vi "AlGaAs_SL_v09.vi"(2 "Debug Mode":bool, 3 "Elapsed Time(s)":dbl, 4 "State":enum16{"Edit", "Start", "Run", "End", "Idle"}(ring), 5 "Argument List In":string[](array[string])) -> (0 "Status Out":string, 1 "Argument List Out":string[](array[string]))   [LabVIEW 2011]
panel:
  out "tPeriod(s)":dbl
  in  "nPeriods":dbl
  out "time array":dbl[](array[numeric])
  out "nPeriod":dbl
  out "tTotal(s) 2":dbl
  out "is_OK":bool
  out "tTotal(s)":dbl
  in  "Tab Control":enum32{"Step 1", "Step 2", "Step 3", "Step 4"}(tab)
  in  "run Ga 1":bool caption="run Ga"
  in  "run Al 1":bool caption="run Al"
  in  "Al flow 1":dbl caption="Al flow(0-100sccm)" format="%.1f"
  in  "time 1":dbl caption="time(s)"
  in  "Ga flow 1":dbl caption="Ga flow(0-10sccm)" format="%.3f"
  in  "run Ga 2":bool caption="run Ga"
  in  "run Al 2":bool caption="run Al"
  in  "Al flow 2":dbl caption="Al flow (0-100sccm)" format="%.1f"
  in  "Ga flow 2":dbl caption="Ga flow (0-10sccm)" format="%.3f"
  in  "time 2":dbl caption="time(s)"
  in  "time 3":dbl caption="time(s)"
  in  "Al flow 3":dbl caption="Al flow (0-100sccm)" format="%.1f"
  in  "run Al 3":bool caption="run Al"
  in  "Ga flow 3":dbl caption="Ga flow (0-10sccm)" format="%.3f"
  in  "run Ga 3":bool caption="run Ga"
  in  "time 4":dbl caption="time(s)"
  in  "Al flow 4":dbl caption="Al flow (0-100sccm)" format="%.1f"
  in  "run Al 4":bool caption="run Al"
  in  "Ga flow 4":dbl caption="Ga flow (0-10sccm)" format="%.3f"
  in  "run Ga 4":bool caption="run Ga"
  out "tphase(s)":dbl[](array[numeric])
  out "phase":i32
  in  "Cancel":bool
  in  "OK":bool
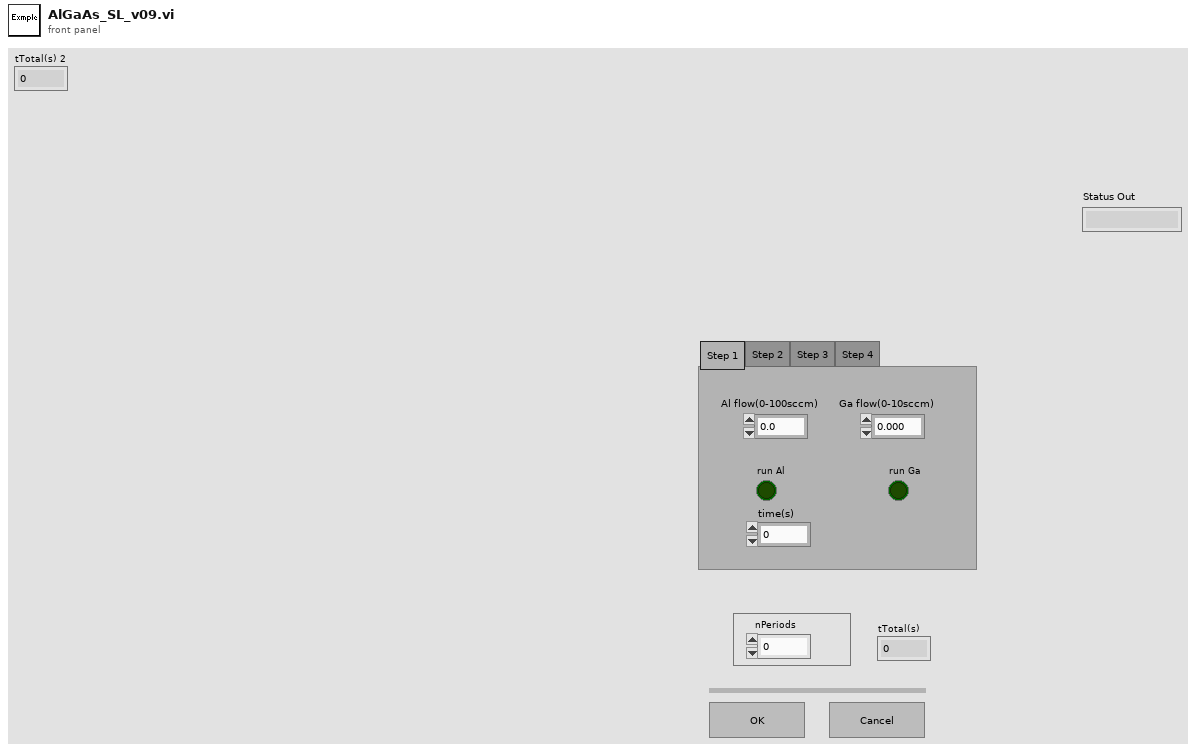
[diagram p1: front panel]
types:
  T1 = enum16{"Discrete", "Continuous", "Instantaneous"}
  T2 = enum32{"Invalid", "Default", "Floating", "Floating/Auto-Hide", "Modal"}
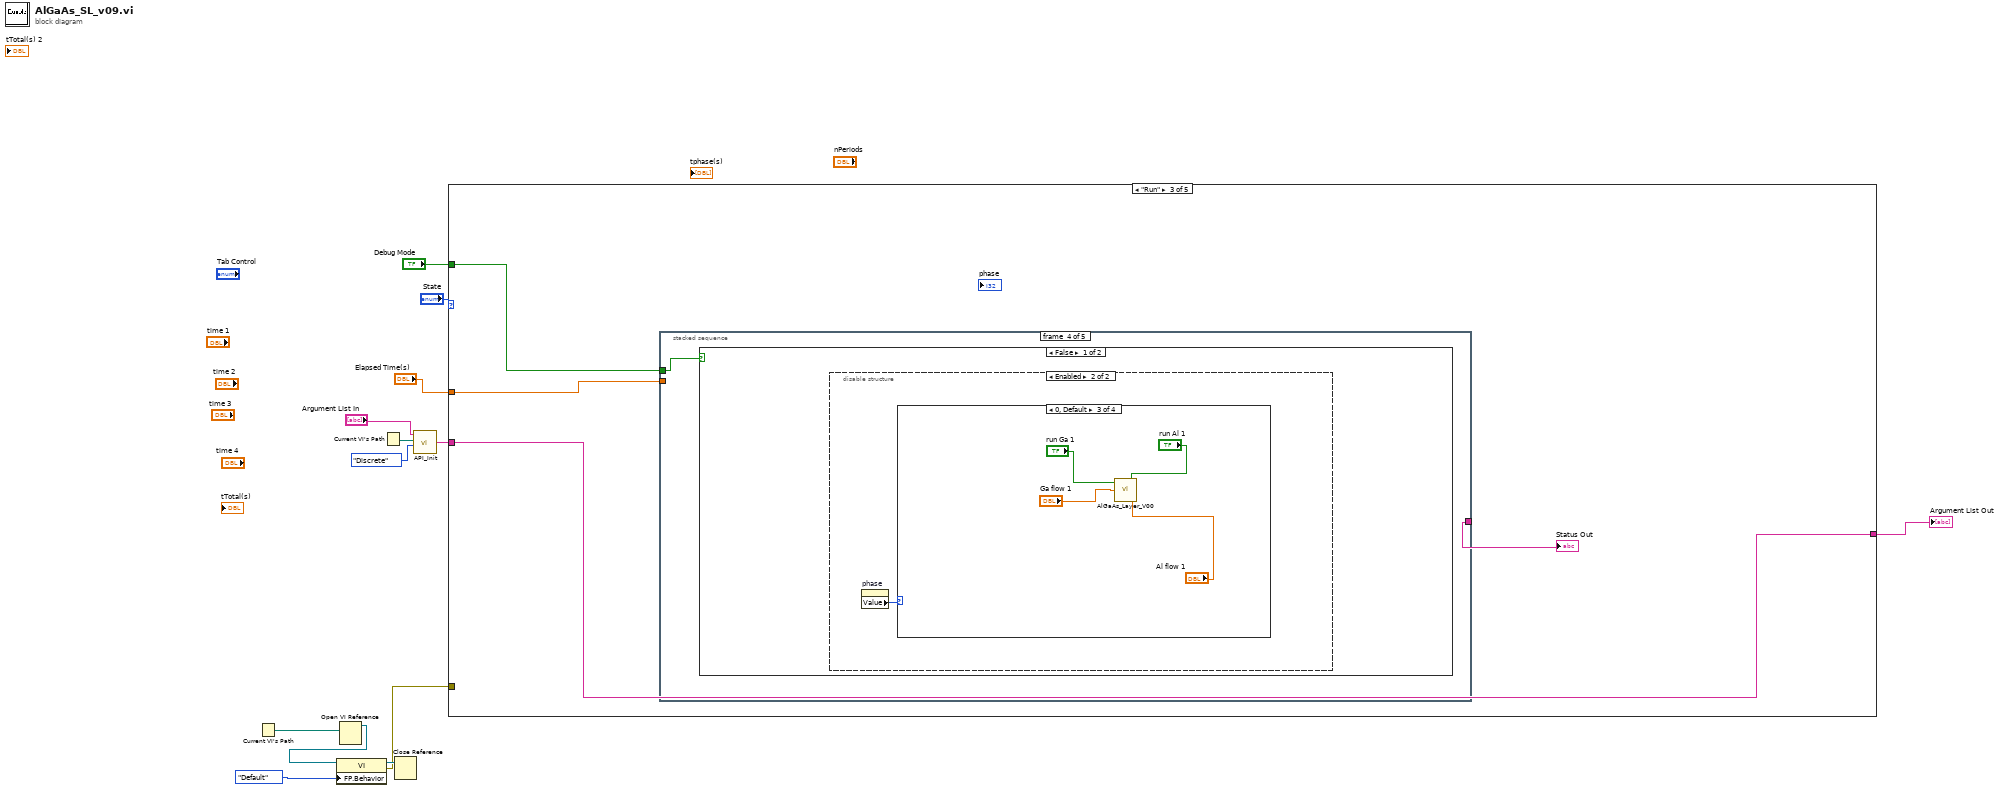
[diagram p0: block diagram]
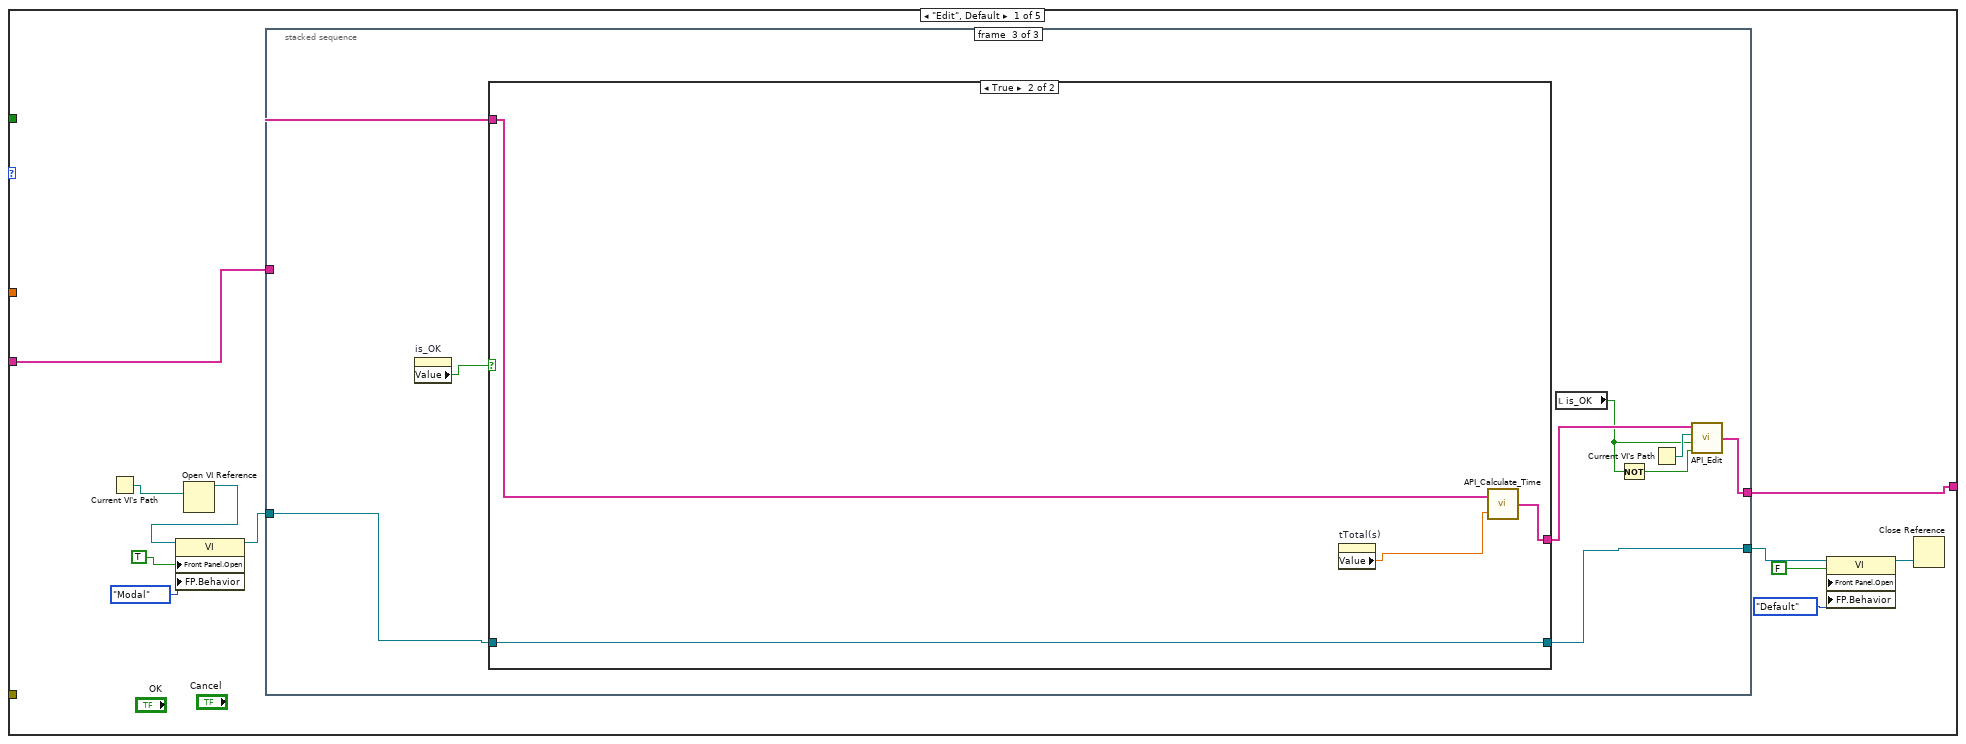
[diagram p2: hidden frame]
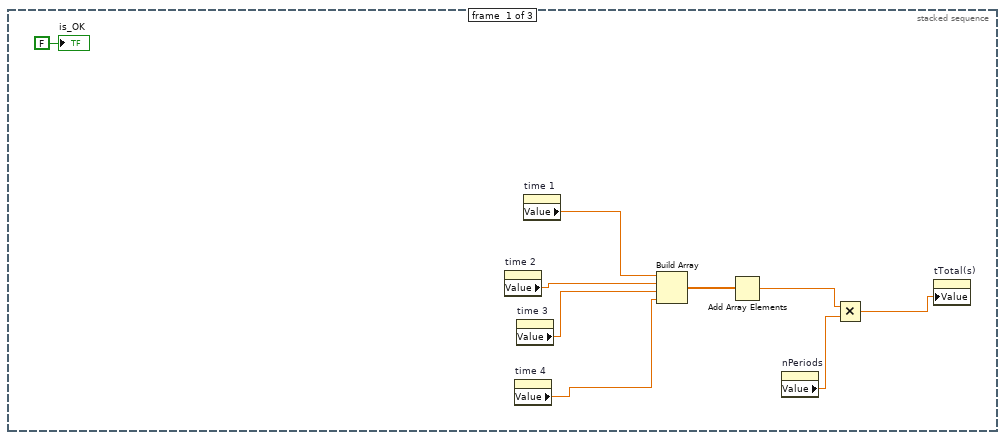
[diagram p3: hidden frame]
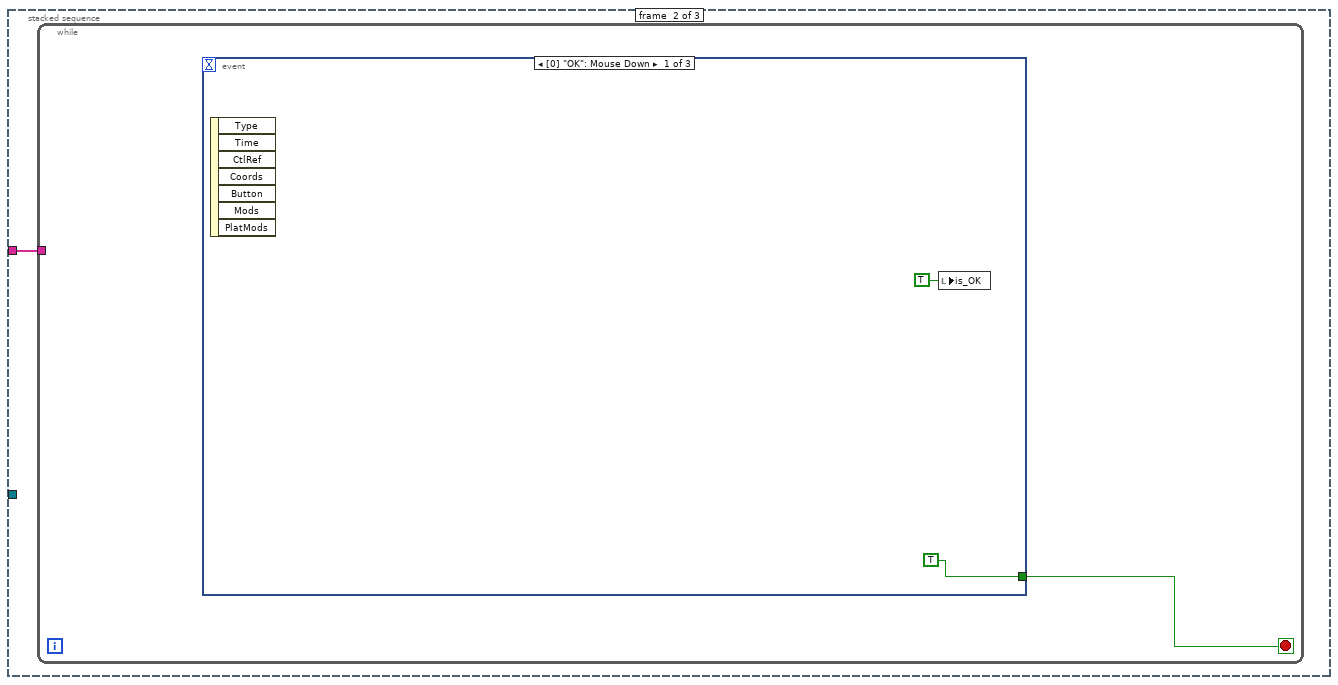
[diagram p4: hidden frame]
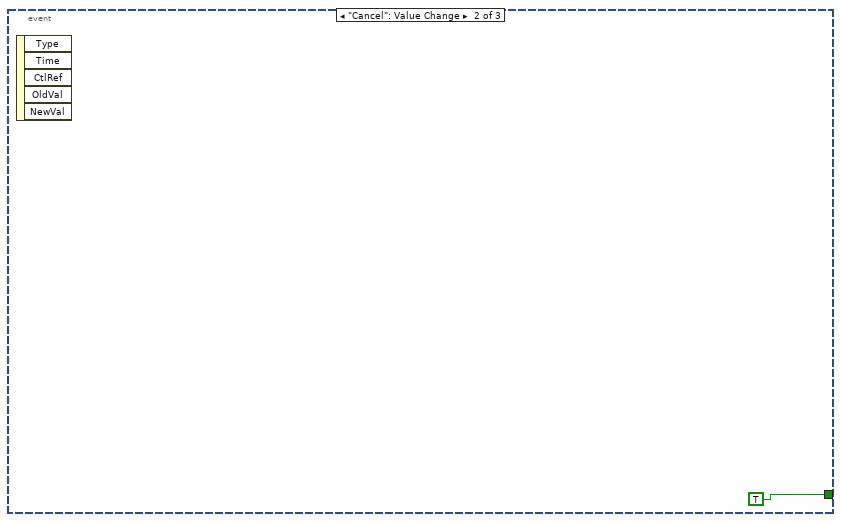
[diagram p5: hidden frame]
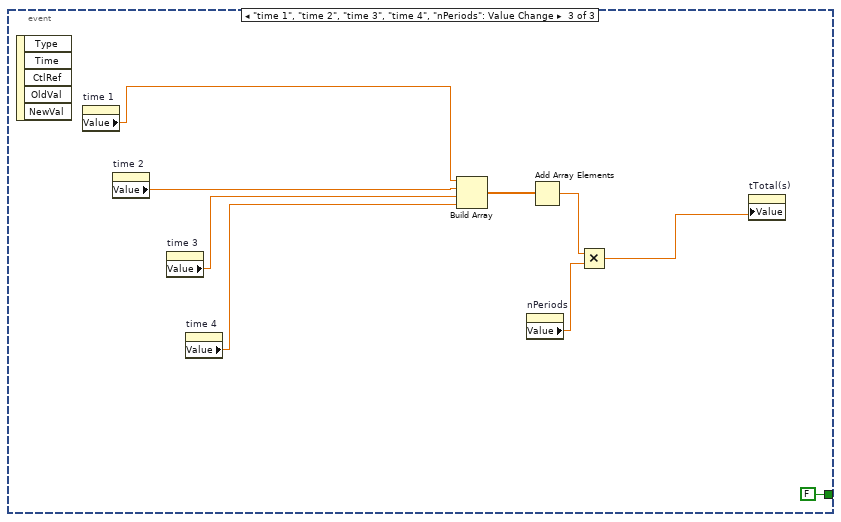
[diagram p6: hidden frame]
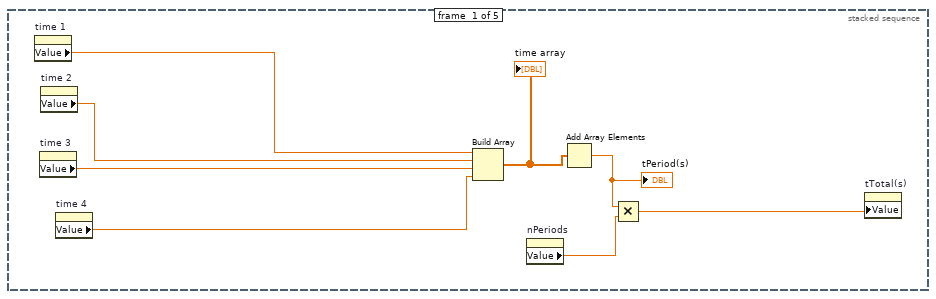
[diagram p9: hidden frame]
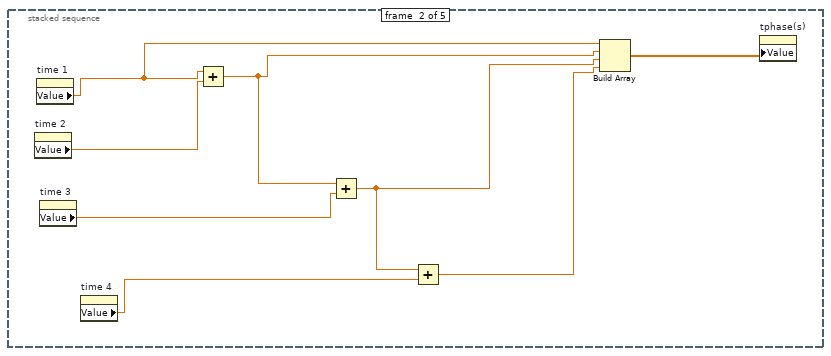
[diagram p10: hidden frame]
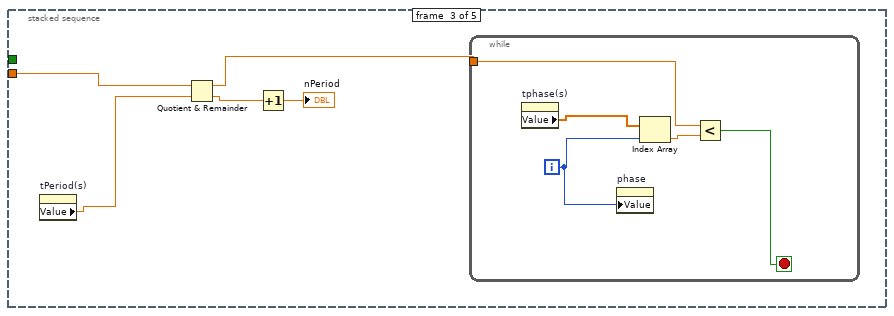
[diagram p11: hidden frame]
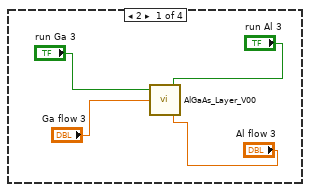
[diagram p13: hidden frame]
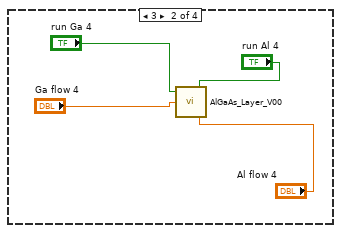
[diagram p14: hidden frame]
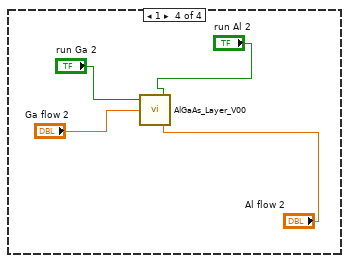
[diagram p15: hidden frame]
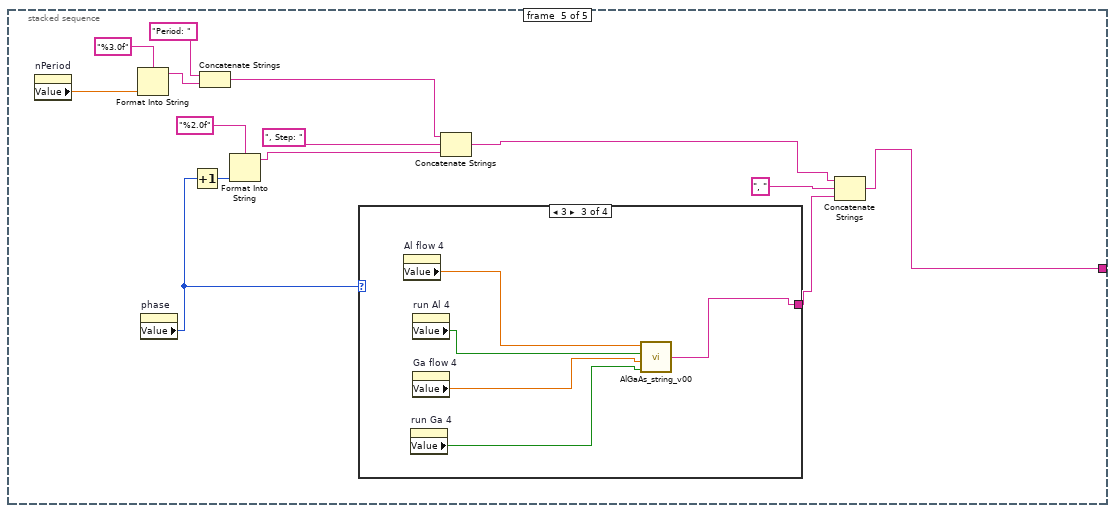
[diagram p17: hidden frame]
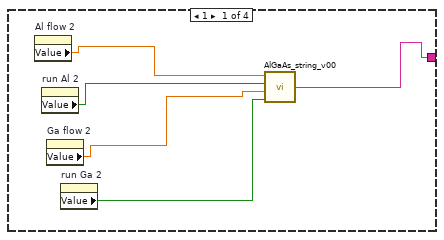
[diagram p18: hidden frame]
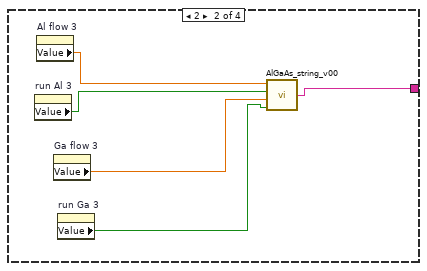
[diagram p19: hidden frame]
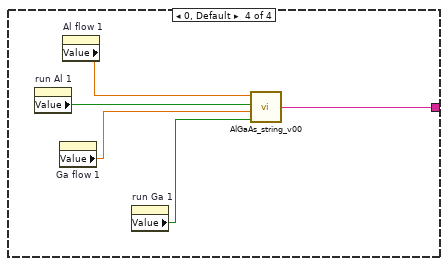
[diagram p20: hidden frame]
diagram:
  n1 = Current VI's Path() -> (path=w9:path)
  n2 = Open VI Reference(vi path=w9) -> (vi reference=w8:refnum<vi>)  [unwired: 1 in, 5 out]
  n3 = property class="VI"(reference=w8, "FP.Behavior"=T2."Default" ("Front Panel Window:Behavior")) -> (reference out=w6:refnum<vi>, error out=w5:errorcluster)  [unwired: 1 in]
  n4 = Current VI's Path() -> (path=w4:path)
  n5 = Close Reference(reference=w6) -> ()  [unwired: 1 in, 1 out]
  n6 = call "API_Init.vi"("API Mode"=T1."Discrete", "VI Path"=w4, "Argument List In"="Argument List In") -> ("Argument List Out"=w1:string[])  [unwired: 1 in]
  n7 = case shown="\"Run\"" "State" {
    tunnel: "Debug Mode" -> [_ _ w66 _ _]
    tunnel: "Elapsed Time(s)" -> [_ _ w67 _ _]
    tunnel: w1 -> [w14 w63 w64 w146 w147]
    tunnel: [w21 w63 w64 w146 w147] -> w10
    tunnel: w5 -> [_ _ _ _ _]
    frame "Edit", Default {
      n8 = Current VI's Path() -> (path=w19:path)
      n9 = Open VI Reference(vi path=w19) -> (vi reference=w18:refnum<vi>)  [unwired: 1 in, 5 out]
      n10 = property class="VI"(reference=w18, "Front Panel.Open"=TRUE ("Front Panel Window:Open"), "FP.Behavior"=T2."Modal" ("Front Panel Window:Behavior")) -> (reference out=w17:refnum<vi>)  [unwired: 1 in, 1 out]
      n11 = stacked-sequence {
        tunnel: w14 -> [_ w34 w56]
        tunnel: w17 -> [_ _ w54]
        tunnel: [_ _ w53] -> w22
        tunnel: [_ _ w50] -> w21
        frame #0 {
          n12 = property on="time 2" class="DigNum (strict)"() -> ("Value"=w30:dbl)  [unwired: 2 in, 2 out]
          n13 = property on="time 4" class="DigNum (strict)"() -> ("Value"=w28:dbl)  [unwired: 2 in, 2 out]
          n14 = property on="time 3" class="DigNum (strict)"() -> ("Value"=w29:dbl)  [unwired: 2 in, 2 out]
          n15 = property on="time 1" class="DigNum (strict)"() -> ("Value"=w32:dbl)  [unwired: 2 in, 2 out]
          n16 = Build Array(w32, w30, w29, w28) -> (w33:dbl[])
          n17 = Add Array Elements(numeric array=w33) -> (sum=w27:dbl)
          n18 = property on="nPeriods" class="DigNum (strict)"() -> ("Value"=w26:dbl)  [unwired: 2 in, 2 out]
          n19 = Multiply(x=w27, y=w26) -> (x*y=w25:dbl)
          n20 = property on="tTotal(s)" class="DigNum (strict)"("Value"=w25) -> ()  [unwired: 2 in, 2 out]
          "is_OK" <- FALSE ("is_OK")
        }
        frame #1 {
          n21 = while {
            tunnel: w34 -> [_]
            stop <- w35 stop-if-true
            n22 = event shown="[0] \"OK\": Mouse Down" {
              selector: _ -> [_ _ _]
              dyn-events: _ -> [_ _ _]
              timeout: _ -> [_ _ _]
              tunnel: [TRUE ("done_editing") TRUE ("done_editing") FALSE ("done_editing")] -> w35
              event "OK": Mouse Down {
                n23 = event-data() -> ()  [unwired: 1 in, 7 out]
                n24 = local write "is_OK"(TRUE ("is_OK")) -> ()
              }
              event "Cancel": Value Change {
                n25 = event-data() -> ()  [unwired: 1 in, 5 out]
              }
              event "time 1", "time 2", "time 3", "time 4", "nPeriods": Value Change {
                n26 = event-data() -> ()  [unwired: 1 in, 5 out]
                n27 = property on="time 1" class="DigNum (strict)"() -> ("Value"=w46:dbl)  [unwired: 2 in, 2 out]
                n28 = property on="time 2" class="DigNum (strict)"() -> ("Value"=w44:dbl)  [unwired: 2 in, 2 out]
                n29 = property on="time 3" class="DigNum (strict)"() -> ("Value"=w43:dbl)  [unwired: 2 in, 2 out]
                n30 = property on="time 4" class="DigNum (strict)"() -> ("Value"=w42:dbl)  [unwired: 2 in, 2 out]
                n31 = Build Array(w46, w44, w43, w42) -> (w45:dbl[])
                n32 = property on="nPeriods" class="DigNum (strict)"() -> ("Value"=w40:dbl)  [unwired: 2 in, 2 out]
                n33 = Add Array Elements(numeric array=w45) -> (sum=w41:dbl)
                n34 = Multiply(x=w41, y=w40) -> (x*y=w39:dbl)
                n35 = property on="tTotal(s)" class="DigNum (strict)"("Value"=w39) -> ()  [unwired: 2 in, 2 out]
              }
            }
          }
        }
        frame #2 {
          n36 = property on="is_OK" class="Bool (strict)"() -> ("Value"=w55:bool)  [unwired: 2 in, 2 out]
          n37 = case shown="True" w55 {
            tunnel: w56 -> [w58 w60]
            tunnel: [w58 w61] -> w51
            tunnel: w54 -> [w57 w62]
            tunnel: [w57 w62] -> w53
            frame False {
            }
            frame True {
              n38 = property on="tTotal(s)" class="DigNum (strict)"() -> ("Value"=w59:dbl)  [unwired: 2 in, 2 out]
              n39 = call "API_Calculate_Time.vi"("Time"=w59, "Argument List In"=w60) -> ("Argument List Out"=w61:string[])
            }
          }
          n40 = local read "is_OK"() -> (w49:bool)
          n41 = Not(x=w49) -> (.not. x?=w48:bool)
          n42 = Current VI's Path() -> (path=w52:path)
          n43 = call "API_Edit.vi"("Cancel"=w48, "OK"=w49, "VI Path"=w52, "Argument List In"=w51) -> ("Argument List Out"=w50:string[])
        }
      }
      n44 = property class="VI"(reference=w22, "Front Panel.Open"=FALSE ("Front Panel Window:Open"), "FP.Behavior"=T2."Default" ("Front Panel Window:Behavior")) -> (reference out=w23:refnum<vi>)  [unwired: 1 in, 1 out]
      n45 = Close Reference(reference=w23) -> ()  [unwired: 1 in, 1 out]
    }
    frame "Start" {
    }
    frame "Run" {
      n46 = stacked-sequence {
        tunnel: w67 -> [_ _ w88 _ _]
        tunnel: w66 -> [_ _ _ w94 _]
        tunnel: [_ _ _ _ w125] -> w65
        frame #0 {
          n47 = property on="time 1" class="DigNum (strict)"() -> ("Value"=w75:dbl)  [unwired: 2 in, 2 out]
          n48 = property on="time 3" class="DigNum (strict)"() -> ("Value"=w73:dbl)  [unwired: 2 in, 2 out]
          n49 = property on="time 2" class="DigNum (strict)"() -> ("Value"=w74:dbl)  [unwired: 2 in, 2 out]
          n50 = property on="time 4" class="DigNum (strict)"() -> ("Value"=w72:dbl)  [unwired: 2 in, 2 out]
          n51 = Build Array(w75, w74, w73, w72) -> (w71:dbl[])
          "time array" <- w71
          n52 = property on="nPeriods" class="DigNum (strict)"() -> ("Value"=w68:dbl)  [unwired: 2 in, 2 out]
          n53 = Add Array Elements(numeric array=w71) -> (sum=w70:dbl)
          "tPeriod(s)" <- w70
          n54 = Multiply(x=w70, y=w68) -> (x*y=w69:dbl)
          n55 = property on="tTotal(s)" class="DigNum (strict)"("Value"=w69) -> ()  [unwired: 2 in, 2 out]
        }
        frame #1 {
          n56 = property on="time 2" class="DigNum (strict)"() -> ("Value"=w81:dbl)  [unwired: 2 in, 2 out]
          n57 = property on="time 1" class="DigNum (strict)"() -> ("Value"=w82:dbl)  [unwired: 2 in, 2 out]
          n58 = property on="time 3" class="DigNum (strict)"() -> ("Value"=w79:dbl)  [unwired: 2 in, 2 out]
          n59 = property on="time 4" class="DigNum (strict)"() -> ("Value"=w77:dbl)  [unwired: 2 in, 2 out]
          n60 = Add(x=w82, y=w81) -> (x+y=w80:dbl)
          n61 = Add(x=w80, y=w79) -> (x+y=w78:dbl)
          n62 = Add(x=w78, y=w77) -> (x+y=w76:dbl)
          n63 = Build Array(w82, w80, w78, w76) -> (w83:dbl[])
          n64 = property on="tphase(s)" class="Arr (strict)"("Value"=w83) -> ()  [unwired: 2 in, 2 out]
        }
        frame #2 {
          n65 = property on="tPeriod(s)" class="DigNum (strict)"() -> ("Value"=w84:dbl)  [unwired: 2 in, 2 out]
          n66 = Quotient & Remainder(x=w88, y=w84) -> (x-y*floor(x/y)=w87:dbl, floor(x/y)=w86:dbl)
          n67 = Increment(x=w86) -> (x+1=→"nPeriod":dbl)
          n68 = while {
            tunnel: w87 -> [w92]
            i -> [w90]
            stop <- w89 stop-if-true
            n69 = property on="tphase(s)" class="Arr (strict)"() -> ("Value"=w93:dbl[])  [unwired: 2 in, 2 out]
            n70 = property on="phase" class="DigNum (strict)"("Value"=w90) -> ()  [unwired: 2 in, 2 out]
            n71 = Index Array(array=w93, index=w90) -> (element=w91:dbl)
            n72 = Less?(x=w92, y=w91) -> (x < y?=w89:bool)
          }
        }
        frame #3 {
          n73 = case shown="False" w94 {
            frame False {
              n74 = disable-structure shown="Enabled" {
                frame Disabled {
                }
                frame Enabled {
                  n75 = property on="phase" class="DigNum (strict)"() -> ("Value"=w95:i32)  [unwired: 2 in, 2 out]
                  n76 = case shown="0, Default" w95 {
                    frame 2 {
                      n77 = call "AlGaAs_Layer_V00.vi"("Aluminum Flow"="Al flow 3", "Al Run"="run Al 3", "Ga flow (0-10 sccm)"="Ga flow 3", "Ga Run"="run Ga 3") -> ()  [unwired: 1 in]
                    }
                    frame 3 {
                      n78 = call "AlGaAs_Layer_V00.vi"("Aluminum Flow"="Al flow 4", "Al Run"="run Al 4", "Ga flow (0-10 sccm)"="Ga flow 4", "Ga Run"="run Ga 4") -> ()  [unwired: 1 in]
                    }
                    frame 0, Default {
                      n79 = call "AlGaAs_Layer_V00.vi"("Aluminum Flow"="Al flow 1", "Al Run"="run Al 1", "Ga flow (0-10 sccm)"="Ga flow 1", "Ga Run"="run Ga 1") -> ()  [unwired: 1 in]
                    }
                    frame 1 {
                      n80 = call "AlGaAs_Layer_V00.vi"("Aluminum Flow"="Al flow 2", "Al Run"="run Al 2", "Ga flow (0-10 sccm)"="Ga flow 2", "Ga Run"="run Ga 2") -> ()  [unwired: 1 in]
                    }
                  }
                }
              }
            }
            frame True {
            }
          }
        }
        frame #4 {
          n81 = property on="nPeriod" class="DigNum (strict)"() -> ("Value"=w117:dbl)  [unwired: 2 in, 2 out]
          n82 = Format Into String(format string="%3.0f", w117) -> (resulting string=w116:string)  [unwired: 2 in, 1 out]
          n83 = property on="phase" class="DigNum (strict)"() -> ("Value"=w119:i32)  [unwired: 2 in, 2 out]
          n84 = Increment(x=w119) -> (x+1=w118:i32)
          n85 = Concatenate Strings("Period: " ("string"), w116) -> (w113:string)
          n86 = Format Into String(format string="%2.0f", w118) -> (resulting string=w123:string)  [unwired: 2 in, 1 out]
          n87 = case shown="3" w119 {
            tunnel: [w126 w131 w136 w145] -> w112
            frame 1 {
              n88 = property on="Al flow 2" class="DigNum (strict)"() -> ("Value"=w130:dbl)  [unwired: 2 in, 2 out]
              n89 = property on="run Al 2" class="Bool (strict)"() -> ("Value"=w129:bool)  [unwired: 2 in, 2 out]
              n90 = property on="Ga flow 2" class="DigNum (strict)"() -> ("Value"=w128:dbl)  [unwired: 2 in, 2 out]
              n91 = property on="run Ga 2" class="Bool (strict)"() -> ("Value"=w127:bool)  [unwired: 2 in, 2 out]
              n92 = call "AlGaAs_string_v00.vi"("Ga run"=w127, "RGa"=w128, "Al run"=w129, "RAl"=w130) -> ("result"=w126:string)
            }
            frame 2 {
              n93 = property on="run Al 3" class="Bool (strict)"() -> ("Value"=w134:bool)  [unwired: 2 in, 2 out]
              n94 = property on="Al flow 3" class="DigNum (strict)"() -> ("Value"=w135:dbl)  [unwired: 2 in, 2 out]
              n95 = property on="Ga flow 3" class="DigNum (strict)"() -> ("Value"=w133:dbl)  [unwired: 2 in, 2 out]
              n96 = property on="run Ga 3" class="Bool (strict)"() -> ("Value"=w132:bool)  [unwired: 2 in, 2 out]
              n97 = call "AlGaAs_string_v00.vi"("Ga run"=w132, "RGa"=w133, "Al run"=w134, "RAl"=w135) -> ("result"=w131:string)
            }
            frame 3 {
              n98 = property on="Al flow 4" class="DigNum (strict)"() -> ("Value"=w140:dbl)  [unwired: 2 in, 2 out]
              n99 = property on="run Ga 4" class="Bool (strict)"() -> ("Value"=w137:bool)  [unwired: 2 in, 2 out]
              n100 = property on="run Al 4" class="Bool (strict)"() -> ("Value"=w139:bool)  [unwired: 2 in, 2 out]
              n101 = property on="Ga flow 4" class="DigNum (strict)"() -> ("Value"=w138:dbl)  [unwired: 2 in, 2 out]
              n102 = call "AlGaAs_string_v00.vi"("Ga run"=w137, "RGa"=w138, "Al run"=w139, "RAl"=w140) -> ("result"=w136:string)
            }
            frame 0, Default {
              n103 = property on="run Al 1" class="Bool (strict)"() -> ("Value"=w142:bool)  [unwired: 2 in, 2 out]
              n104 = property on="Ga flow 1" class="DigNum (strict)"() -> ("Value"=w143:dbl)  [unwired: 2 in, 2 out]
              n105 = property on="Al flow 1" class="DigNum (strict)"() -> ("Value"=w144:dbl)  [unwired: 2 in, 2 out]
              n106 = property on="run Ga 1" class="Bool (strict)"() -> ("Value"=w141:bool)  [unwired: 2 in, 2 out]
              n107 = call "AlGaAs_string_v00.vi"("Ga run"=w141, "RGa"=w143, "Al run"=w142, "RAl"=w144) -> ("result"=w145:string)
            }
          }
          n108 = Concatenate Strings(w113, ", Step: " ("string"), w123) -> (w121:string)
          n109 = Concatenate Strings(w121, ", " ("string"), w112) -> (w125:string)
        }
      }
      "Status Out" <- w65
    }
    frame "End" {
    }
    frame "Idle" {
    }
  }
  "Argument List Out" <- w10
